vi "epx_Vector_Arrow.vi"(9 "Arrow Type":u32, 11 "Phasor":cdb) -> (3 "Vector Arow":cluster{dbl[], dbl[]})   [LabVIEW 2011, in "NI_EP_Basic.lvlib" / "EPX Vector Diagram.xctl"]
uses:
  <vilib>/addons/Electrical Power/Basic/Controls/Vector Diagram/EPX Vector Diagram.xctl
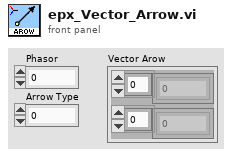
[diagram p1: front panel]
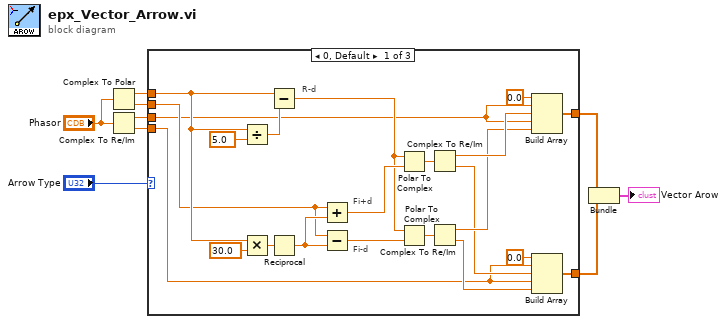
[diagram p0: block diagram]
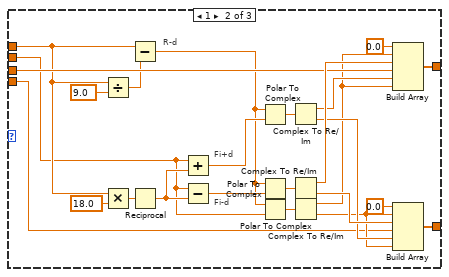
[diagram p2: hidden frame]
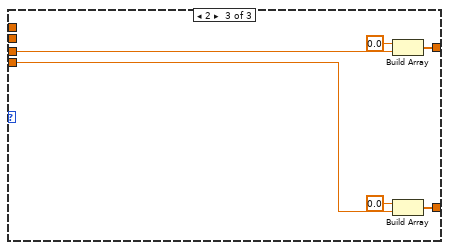
[diagram p3: hidden frame]
diagram:
  n1 = Complex To Polar(r * e^(i*theta)="Phasor") -> (r=w5:dbl, theta=w9:dbl)
  n2 = Complex To Re/Im(x + iy="Phasor") -> (x=w3:dbl, y=w2:dbl)
  n3 = case shown="0, Default" "Arrow Type" {
    tunnel: w5 -> [w20 w38 _]
    tunnel: w9 -> [w19 w34 _]
    tunnel: w3 -> [w11 w43 w58]
    tunnel: w2 -> [w10 w32 w57]
    tunnel: [w17 w40 w60] -> w8
    tunnel: [w16 w39 w59] -> w7
    frame 0, Default {
      # "R-d"
      # "Fi-d"
      # "Fi+d"
      n4 = Divide(x=w20, y=5.0 ("UpravaR")) -> (x/y=w13:dbl)
      n5 = Multiply(x=w20, y=30.0 ("Uprava Fi")) -> (x*y=w27:dbl)
      n6 = Subtract(x=w20, y=w13) -> (x-y=w12:dbl)
      n7 = Reciprocal(x=w27) -> (1/x=w28:dbl)
      n8 = Add(x=w19, y=w28) -> (x+y=w29:dbl)
      n9 = Subtract(x=w19, y=w28) -> (x-y=w31:dbl)
      n10 = Polar To Complex(1:w29, 2:w12) -> (0:w26:cdb)
      n11 = Polar To Complex(1:w31, 2:w12) -> (0:w30:cdb)
      n12 = Complex To Re/Im(x + iy=w26) -> (x=w23:dbl, y=w18:dbl)
      n13 = Complex To Re/Im(x + iy=w30) -> (x=w21:dbl, y=w22:dbl)
      n14 = Build Array(0.0 ("element"), w11, w23, w11, w21) -> (w17:dbl[])
      n15 = Build Array(0.0 ("element"), w10, w18, w10, w22) -> (w16:dbl[])
    }
    frame 1 {
      # "R-d"
      # "Fi+d"
      # "Fi-d"
      n16 = Divide(x=w38, y=9.0 ("UpravaR")) -> (x/y=w36:dbl)
      n17 = Multiply(x=w38, y=18.0 ("Uprava Fi")) -> (x*y=w52:dbl)
      n18 = Subtract(x=w38, y=w36) -> (x-y=w35:dbl)
      n19 = Reciprocal(x=w52) -> (1/x=w53:dbl)
      n20 = Add(x=w34, y=w53) -> (x+y=w54:dbl)
      n21 = Subtract(x=w34, y=w53) -> (x-y=w56:dbl)
      n22 = Polar To Complex(1:w54, 2:w35) -> (0:w51:cdb)
      n23 = Polar To Complex(1:w56, 2:w35) -> (0:w55:cdb)
      n24 = Polar To Complex(1:w34, 2:w35) -> (0:w49:cdb)
      n25 = Complex To Re/Im(x + iy=w51) -> (x=w46:dbl, y=w45:dbl)
      n26 = Complex To Re/Im(x + iy=w55) -> (x=w48:dbl, y=w47:dbl)
      n27 = Complex To Re/Im(x + iy=w49) -> (x=w33:dbl, y=w44:dbl)
      n28 = Build Array(0.0 ("element"), w33, w48, w43, w46, w33) -> (w40:dbl[])
      n29 = Build Array(0.0 ("element"), w44, w47, w32, w45, w44) -> (w39:dbl[])
    }
    frame 2 {
      n30 = Build Array(0.0 ("element"), w58) -> (w60:dbl[])
      n31 = Build Array(0.0 ("element"), w57) -> (w59:dbl[])
    }
  }
  n32 = Bundle ("Ia")(w8, w7) -> (→"Vector Arow":cluster{dbl[], dbl[]})  [unwired: 1 in]
